vi "sub_vi_prompt_calibration_weights.vi"(2 "Title":string) -> (16 "Weights number 2":dbl)   [LabVIEW 2016]
doc: "Displays a standard dialog box that prompts users to enter information, such as a user name and password.\n--------------------\n\nThis Express VI is configured as follows:\n\nMessage to Display to the User:\nThe inputs are: \nNumber: tttt"
panel:
  in  "OK Button":bool
  in  "Weights number":dbl min=0.0 step=1.0
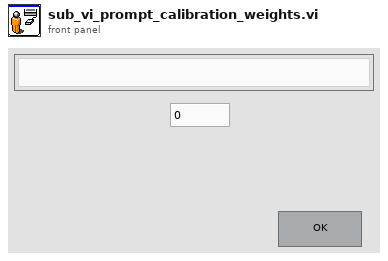
[diagram p1: front panel]
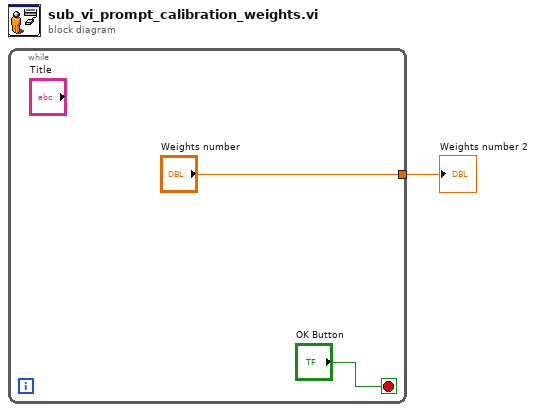
[diagram p0: block diagram]
diagram:
  n1 = while {
    tunnel: ["Weights number"] -> w1
    stop <- "OK Button" stop-if-true
  }
  "Weights number 2" <- w1
